vi "Write pyCmdSession.vi"(8 "error in (no error)":errorcluster, 10 "pyCmdSession":refnum<k35>, 11 "pyCode in":refnum<class "pyCode.lvclass">) -> (0 "error out":errorcluster, 3 "pyCode out":refnum<class "pyCode.lvclass">)   [LabVIEW 2018, in "pyCode.lvclass"]
uses:
  pyCode.lvclass
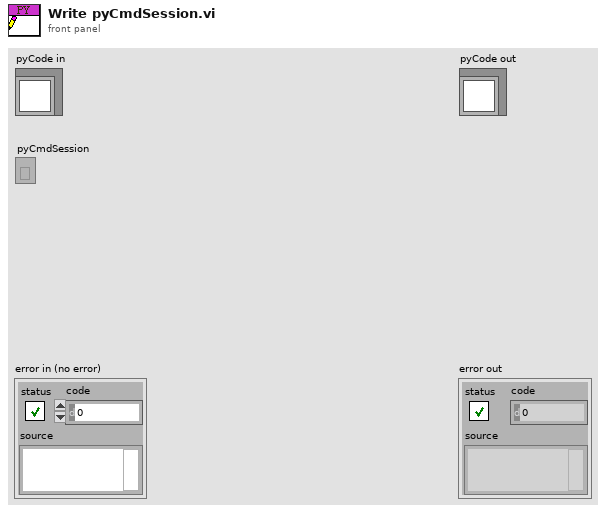
[diagram p1: front panel]
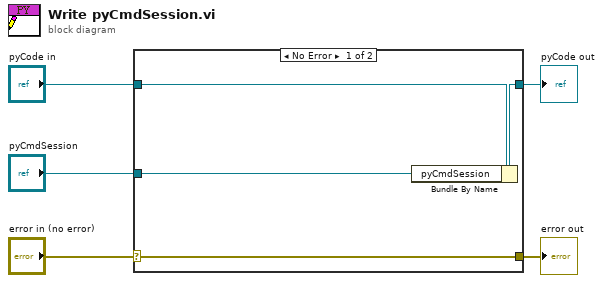
[diagram p0: block diagram]
diagram:
  n1 = case shown="No Error" "error in (no error)" {
    selector: "error in (no error)" -> [w9 w10]
    tunnel: [w9 w10] -> w4
    tunnel: [w7 w11] -> w2
    tunnel: "pyCode in" -> [w8 w11]
    tunnel: "pyCmdSession" -> [w6 _]
    frame No Error {
      n2 = Bundle By Name(cluster=w8, "pyCmdSession"=w6) -> (w7:refnum<class "pyCode.lvclass">)
    }
    frame Error {
    }
  }
  "error out" <- w4
  "pyCode out" <- w2
